vi "Add Random Colors to Edges.vi"(11 "Graph in":refnum<class "Graph.lvclass">) -> (3 "Graphviz out":refnum<class "Graphviz.lvclass">)   [LabVIEW 2020, in "SimpleDependencyInspector.lvlib"]
uses:
  SimpleDependencyInspector.lvlib
  <vilib>/GraphBuilder/Graph/Graph.lvclass
  <vilib>/GraphBuilder/Renderer/Graphviz/Graphviz.lvclass
  <vilib>/GraphBuilder/Renderer/Graphviz/Graph Direction.ctl
  <vilib>/GraphBuilder/Renderer/Graphviz/Specific Edge Shape Def.ctl
  <vilib>/GraphBuilder/Shapes/Edge/Graphviz/Graphviz Edge Shape.lvclass
  <vilib>/GraphBuilder/Edge/Edge.lvclass
  <vilib>/GraphBuilder/Shapes/Edge/Graphviz/Shape.ctl
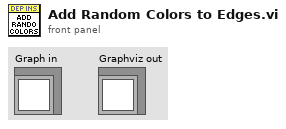
[diagram p1: front panel]
types:
  T1 = typedef "GraphBuilder.lvlib/Graphviz.lvclass/Graph Direction.ctl" = enum16{"Top to Bottom", "Left To Right", "Bottom to Top", "Right to Left"}
  T2 = typedef "GraphBuilder.lvlib/Graphviz Edge Shape.lvclass/Shape.ctl" = enum16{"box", "lbox", "rbox", "obox", "olbox", "orbox", "crow", "lcrow", "rcrow", "diamond", "ldiamond", "rdiamond", "odiamond", "oldiamond", "ordiamond", "dot", "odot", "inv", "linv", "rinv", "oinv", "olinv", "orinv", "none", "normal", "lnormal", "rnormal", "onormal", "olnormal", "ornormal", "tee", "ltee", "rtee", "vee", "lvee", "rvee", "curve", "lcurve", "rcurve", "icurve", "licurve", "ricurve"}
  T3 = typedef "GraphBuilder.lvlib/Graphviz.lvclass/Specific Edge Shape Def.ctl" = cluster{"Graphviz Edge Shape":refnum<class "Graphviz Edge Shape.lvclass">, "Edge":refnum<class "Edge.lvclass">}
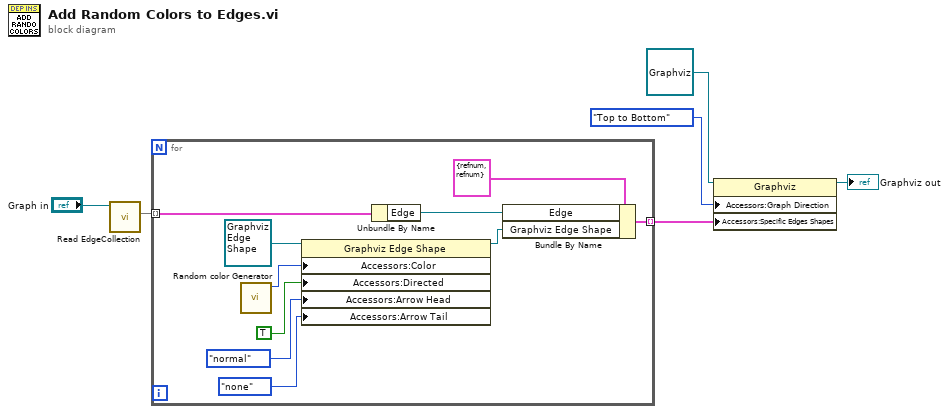
[diagram p0: block diagram]
diagram:
  n1 = call-dynamic "Read EdgeCollection.vi"("Graph in"="Graph in") -> ("EdgeCollection"=w5:map{string, refnum<class "Edge.lvclass">})  [unwired: 9 in, 1 out]
  n2 = for {
    tunnel: w5 -> [w10] mode=indexing
    tunnel: [w8] -> w6 mode=indexing
    n3 = call "Random color Generator.vi"() -> ("Random Color"=w7:i64)  [unwired: 11 in]
    n4 = property class="Graphviz Edge Shape"(reference=refnum<class "Graphviz Edge Shape.lvclass"> refnum ("GraphBuilder.lvlib:Graphviz Edge Shape.lvclass"), "Accessors:Color"=w7, "Accessors:Directed"=TRUE ("Directed"), "Accessors:Arrow Head"=Shape."normal" ("Arrow Head"), "Accessors:Arrow Tail"=Shape."none" ("Arrow Tail")) -> (reference out=w12:refnum<class "Graphviz Edge Shape.lvclass">)  [unwired: 1 in, 1 out]
    n5 = Unbundle By Name(w10) -> ("Edge"=w9:refnum<class "Edge.lvclass">)
    n6 = Bundle By Name(cluster=T3 {"Graphviz Edge Shape"=refnum, "Edge"=refnum} ("Specific Node Shape"), "Edge"=w9, "Graphviz Edge Shape"=w12) -> (w8:T3)
  }
  n7 = property class="Graphviz"(reference=refnum<class "Graphviz.lvclass"> refnum ("GraphBuilder.lvlib:Graphviz.lvclass"), "Accessors:Graph Direction"=Graph_Direction."Top to Bottom" ("Graph Direction"), "Accessors:Specific Edges Shapes"=w6) -> (reference out=→"Graphviz out":refnum<class "Graphviz.lvclass">)  [unwired: 1 in, 1 out]
